vi "Rising Edge.vi"(9 "input":bool, 10 "error in":errorcluster) -> (1 "output":bool, 2 "error out":errorcluster)   [LabVIEW 2014]
uses:
  <vilib>/functionblocks/FB Core/FB Core.xnode
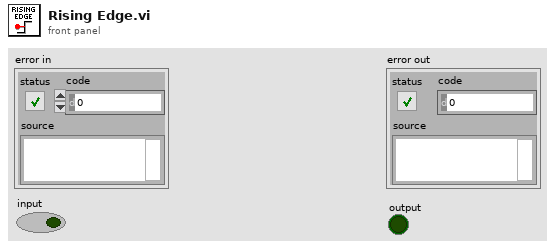
[diagram p1: front panel]
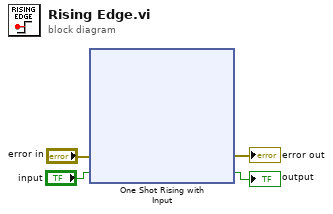
[diagram p0: block diagram]
diagram:
  n1 = xnode "One Shot Rising with Input"("error in"="error in", "input"="input") -> ("error out"=→"error out":errorcluster, "output"=→"output":bool)
